vi "RSOHLayerGen.vi"(6 "Layer":u32=160, 9 "OHpows":dbl[](array[numeric]), 10 "HatchPow":T6={"Power"=300.0, "Mark Speed"=400.0, "Jump Speed"=1000.0}, 11 "RectHatch":T7={"Width"=10.0, "Height"=10.0, "Angle"=45.0, "OffX"=0.1, "OffY"=0.1, "Spacing"=0.1, "IslandSize"=0.1} {"IslandSize" format="%#_13g"; "Spacing" format="%#_13g"; "OffY" format="%#_13g"; "OffX" format="%#_13g"; "Height" format="%#_13g"; "Width" format="%#_13g"}) -> (1 "Hatches2":T1(array[cluster]), 2 "Hatches":T1(array[cluster]), 3 "PathSups":T2[](array[typedef]))   [LabVIEW 2014]
uses:
  TypeDefs/RectHatch.ctl
  TypeDefs/PowerSpeed.ctl
  TypeDefs/PathSupreme.ctl
  PSup2SCAN/Sub/VelocityProfile.ctl
  PSup2SCAN/Sub/PathCut.ctl
  PSup2SCAN/Sub/Segment.ctl
  PSup2SCAN/Sub/Point.ctl
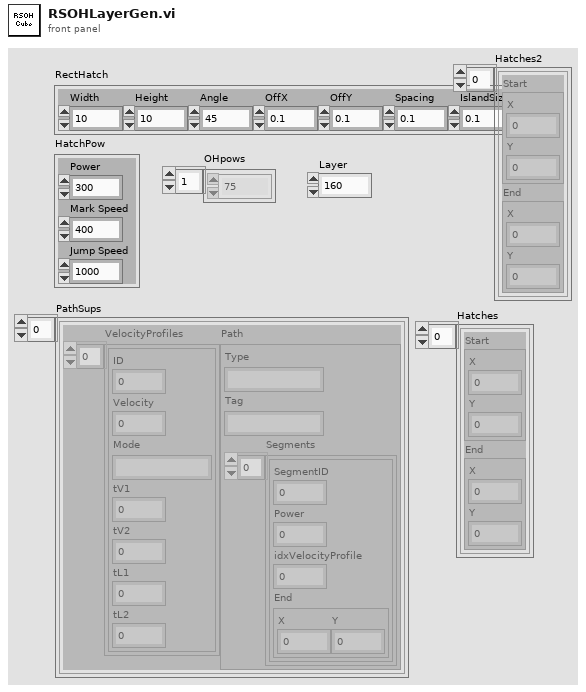
[diagram p1: front panel]
types:
  T1 = cluster{"Start":cluster{"X":dbl, "Y":dbl}, "End":cluster{"X":dbl, "Y":dbl}}[]
  T2 = typedef "PathSupreme.ctl" = cluster{"VelocityProfiles":T3[], "Path":T4}
  T3 = typedef "VelocityProfile.ctl" = cluster{"ID":u32, "Velocity":dbl, "Mode":string, "tV1":u32, "tV2":u32, "tL1":u32, "tL2":u32}
  T4 = typedef "PathCut.ctl" = cluster{"Type":string, "Tag":string, "Segments":T5[]}
  T5 = typedef "Segment.ctl" = cluster{"SegmentID":u16, "Power":sgl, "idxVelocityProfile":u16, "End":cluster{"X":sgl, "Y":sgl}}
  T6 = typedef "PowerSpeed.ctl" = cluster{"Power":dbl, "Mark Speed":dbl, "Jump Speed":dbl}
  T7 = typedef "RectHatch.ctl" = cluster{"Width":dbl, "Height":dbl, "Angle":sgl, "OffX":dbl, "OffY":dbl, "Spacing":dbl, "IslandSize":dbl}
  T8 = typedef "Point.ctl" = cluster{"X":dbl, "Y":dbl}
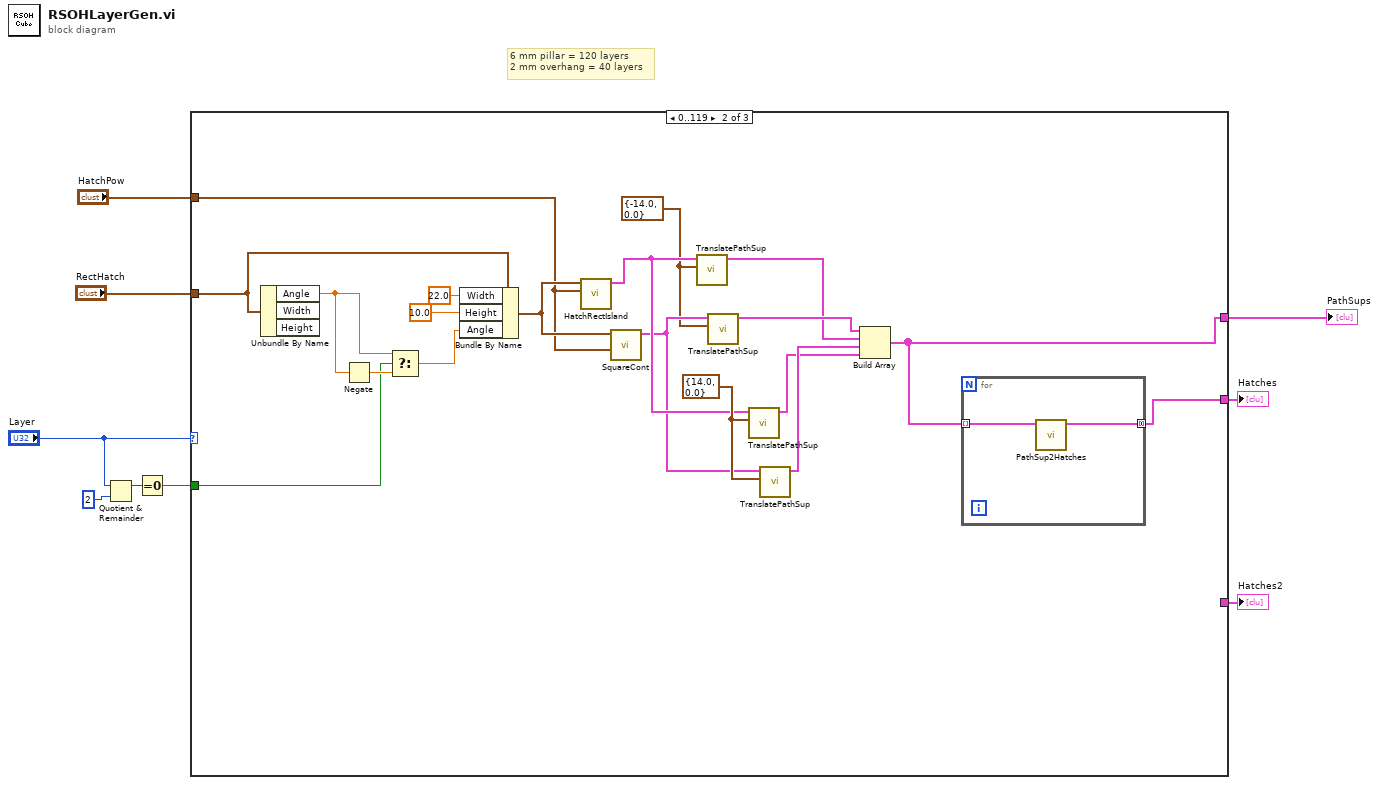
[diagram p0: block diagram]
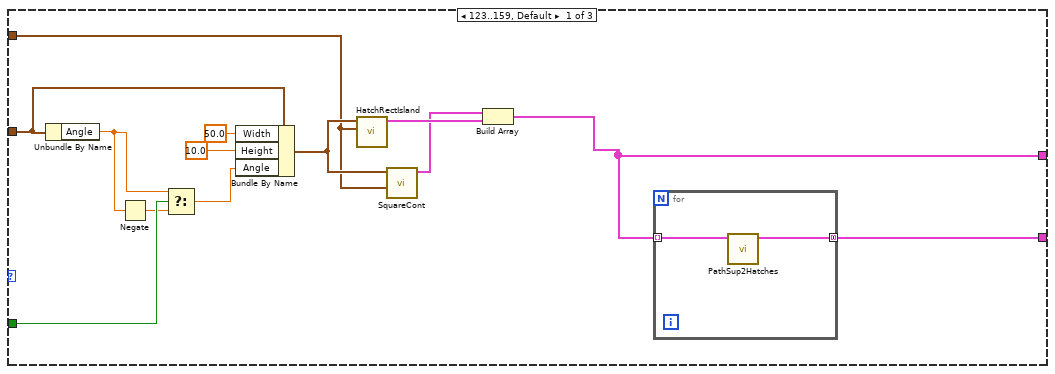
[diagram p2: hidden frame]
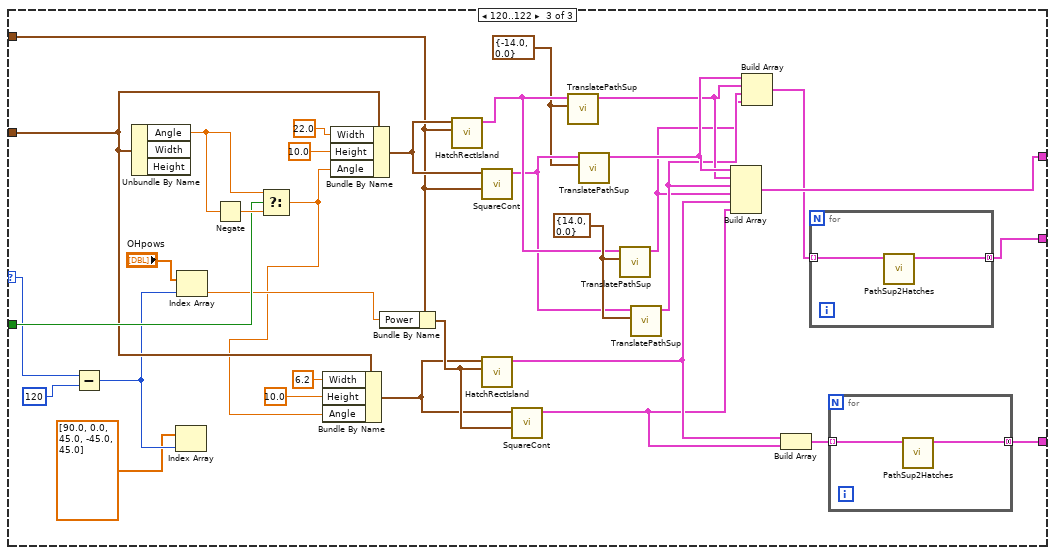
[diagram p3: hidden frame]
diagram:
  # "6 mm pillar = 120 layers\n2 mm overhang = 40 layers"
  n1 = Quotient & Remainder(x="Layer", y=u8 2) -> (x-y*floor(x/y)=w9:u32)  [unwired: 1 out]
  n2 = Equal To 0?(x=w9) -> (x = 0?=w6:bool)
  n3 = case shown="0..119" "Layer" {
    selector: "Layer" -> [_ _ w61]
    tunnel: w6 -> [w22 w38 w72]
    tunnel: "RectHatch" -> [w13 w37 w69]
    tunnel: "HatchPow" -> [w17 w39 w71]
    tunnel: [w12 w28 w65] -> w3
    tunnel: [w14 w27 w53] -> w2
    tunnel: [_ _ w49] -> w1
    frame 123..159, Default {
      n4 = Unbundle By Name(w13) -> ("Angle"=w20:sgl)
      n5 = Negate(x=w20) -> (-x=w21:sgl)
      n6 = Select(t=w20, s=w22, f=w21) -> (s? t:f=w19:sgl)
      n7 = Bundle By Name(cluster=w13, "Width"=50.0, "Height"=10.0, "Angle"=w19) -> (w18:T7)
      n8 = call "HatchRectIsland.vi"("HatchPow"=w17, "RectHatch"=w18) -> ("PathSupreme"=w16:T2)  [unwired: 9 in]
      n9 = call "SquareCont.vi"("ContPow"=w17, "RectHatch"=w18) -> ("PathSupreme"=w15:T2)  [unwired: 9 in]
      n10 = Build Array(w15, w16) -> (w12:T2[])
      n11 = for {
        tunnel: w12 -> [w24] mode=indexing
        tunnel: [w23] -> w14 mode=concatenating
        n12 = call "PathSup2Hatches.vi"("PathSupOut"=w24) -> ("Hatches"=w23:T1)  [unwired: 10 in]
      }
    }
    frame 0..119 {
      w33 = T8 {"X"=-14.0, "Y"=0.0} ("Offset")
      w36 = T8 {"X"=14.0, "Y"=0.0} ("Offset")
      n13 = Unbundle By Name(w37) -> ("Angle"=w42:sgl)  [unwired: 2 out]
      n14 = Negate(x=w42) -> (-x=w43:sgl)
      n15 = Select(t=w42, s=w38, f=w43) -> (s? t:f=w41:sgl)
      n16 = Bundle By Name(cluster=w37, "Width"=22.0, "Height"=10.0, "Angle"=w41) -> (w40:T7)
      n17 = call "HatchRectIsland.vi"("HatchPow"=w39, "RectHatch"=w40) -> ("PathSupreme"=w35:T2)  [unwired: 9 in]
      n18 = call "SquareCont.vi"("ContPow"=w39, "RectHatch"=w40) -> ("PathSupreme"=w34:T2)  [unwired: 9 in]
      n19 = call "TranslatePathSup.vi"("Offset"=w33, "PathSupreme"=w35) -> ("PathSupOut"=w31:T2)  [unwired: 9 in]
      n20 = call "TranslatePathSup.vi"("Offset"=w33, "PathSupreme"=w34) -> ("PathSupOut"=w32:T2)  [unwired: 9 in]
      n21 = call "TranslatePathSup.vi"("Offset"=w36, "PathSupreme"=w35) -> ("PathSupOut"=w29:T2)  [unwired: 9 in]
      n22 = call "TranslatePathSup.vi"("Offset"=w36, "PathSupreme"=w34) -> ("PathSupOut"=w30:T2)  [unwired: 9 in]
      n23 = Build Array(w32, w31, w30, w29) -> (w28:T2[])
      n24 = for {
        tunnel: w28 -> [w45] mode=indexing
        tunnel: [w44] -> w27 mode=concatenating
        n25 = call "PathSup2Hatches.vi"("PathSupOut"=w45) -> ("Hatches"=w44:T1)  [unwired: 10 in]
      }
    }
    frame 120..122 {
      w73 = T8 {"X"=-14.0, "Y"=0.0} ("Offset")
      w76 = T8 {"X"=14.0, "Y"=0.0} ("Offset")
      n26 = Subtract(x=w61, y=u32 120) -> (x-y=w60:u32)
      n27 = Unbundle By Name(w69) -> ("Angle"=w78:sgl)  [unwired: 2 out]
      n28 = Index Array(array=dbl[] [90.0, 0.0, 45.0, -45.0, 45.0], index=w60) -> ()  [unwired: 1 out]
      n29 = Index Array(array="OHpows", index=w60) -> (element=w63:dbl)
      n30 = Negate(x=w78) -> (-x=w79:sgl)
      n31 = Select(t=w78, s=w72, f=w79) -> (s? t:f=w48:sgl)
      n32 = Bundle By Name(cluster=w69, "Width"=6.2, "Height"=10.0, "Angle"=w48) -> (w66:T7)
      n33 = Bundle By Name(cluster=w69, "Width"=22.0, "Height"=10.0, "Angle"=w48) -> (w77:T7)
      n34 = Bundle By Name(cluster=w71, "Power"=w63) -> (w70:T6)
      n35 = call "HatchRectIsland.vi"("HatchPow"=w71, "RectHatch"=w77) -> ("PathSupreme"=w75:T2)  [unwired: 9 in]
      n36 = call "SquareCont.vi"("ContPow"=w71, "RectHatch"=w77) -> ("PathSupreme"=w74:T2)  [unwired: 9 in]
      n37 = call "HatchRectIsland.vi"("HatchPow"=w70, "RectHatch"=w66) -> ("PathSupreme"=w52:T2)  [unwired: 9 in]
      n38 = call "SquareCont.vi"("ContPow"=w70, "RectHatch"=w66) -> ("PathSupreme"=w51:T2)  [unwired: 9 in]
      n39 = call "TranslatePathSup.vi"("Offset"=w73, "PathSupreme"=w75) -> ("PathSupOut"=w57:T2)  [unwired: 9 in]
      n40 = call "TranslatePathSup.vi"("Offset"=w73, "PathSupreme"=w74) -> ("PathSupOut"=w58:T2)  [unwired: 9 in]
      n41 = call "TranslatePathSup.vi"("Offset"=w76, "PathSupreme"=w75) -> ("PathSupOut"=w55:T2)  [unwired: 9 in]
      n42 = call "TranslatePathSup.vi"("Offset"=w76, "PathSupreme"=w74) -> ("PathSupOut"=w56:T2)  [unwired: 9 in]
      n43 = Build Array(w58, w57, w56, w55, w52, w51) -> (w65:T2[])
      n44 = Build Array(w58, w57, w56, w55) -> (w54:T2[])
      n45 = Build Array(w52, w51) -> (w50:T2[])
      n46 = for {
        tunnel: w54 -> [w83] mode=indexing
        tunnel: [w82] -> w53 mode=concatenating
        n47 = call "PathSup2Hatches.vi"("PathSupOut"=w83) -> ("Hatches"=w82:T1)  [unwired: 10 in]
      }
      n48 = for {
        tunnel: w50 -> [w81] mode=indexing
        tunnel: [w80] -> w49 mode=concatenating
        n49 = call "PathSup2Hatches.vi"("PathSupOut"=w81) -> ("Hatches"=w80:T1)  [unwired: 10 in]
      }
    }
  }
  "PathSups" <- w3
  "Hatches" <- w2
  "Hatches2" <- w1
